vi "Day 19-Apply Transformation.vi"(9 "3D LinearOffset":i32[](array[numeric]), 10 "Rotation":T1, 11 "Point in":i32[](array[numeric])) -> (3 "Point out":i32[](array[numeric]))   [LabVIEW 2021]
uses:
  <vilib>/Analysis/Matrix/NI_Matrix.lvlib
  <vilib>/Analysis/Matrix/Numeric/Conversions/Matrix To Array - RM.vi
  <vilib>/Analysis/Matrix/Numeric/Multiply/Multiply - RM,RM.vi
  <vilib>/Analysis/Matrix/Numeric/Conversions/Array To Matrix - RA.vi
  <vilib>/Analysis/Matrix/Datatypes/RealMatrix.ctl
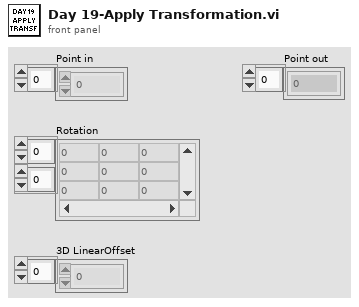
[diagram p1: front panel]
types:
  T1 = typedef "NI_Matrix.lvlib/RealMatrix.ctl" = dbl[][]
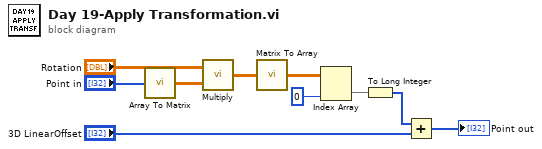
[diagram p0: block diagram]
diagram:
  n1 = call-poly <vilib>:"Array To Matrix.vi"("Real 1D Array"="Point in") -> ("Real Matrix (Column Vector)"=w3:T1)
  n2 = call-poly <vilib>:"Multiply.vi"("Real Matrix B"=w3, "Real Matrix A"="Rotation") -> ("A * B"=w4:T1)
  n3 = call-poly <vilib>:"Matrix To Array.vi"("Real Matrix"=w4) -> ("Real 2D Array"=w5:dbl[][])
  n4 = Index Array(array=w5, index (col)=0 ("disabled index (col)")) -> (element=w7:dbl[])  [unwired: 1 in]
  n5 = To Long Integer(number=w7) -> (32bit integer=w9:i32[])
  n6 = Add(x=w9, y="3D LinearOffset") -> (x+y=→"Point out":i32[])
